vi "FileAscOpen.vi"(6 "提示语":refnum<vi>, 7 "Language":u32, 8 "进度条":refnum<vi>, 9 "进度数值":refnum<vi>, 10 "报文行数统计":refnum<vi>, 11 "file path (dialog if empty)":path caption="文件路径 （空时为对话框）") -> (0 "路径输出":path, 1 "重构的Data数组":u32[][](array[numeric]), 2 "统计数量":string[](array[string]), 3 "报文ID":string[](array[string]), 4 "基时间簇":T1 {"基时间秒" format="%#.6f"}, 5 "CAN报文统计":string[][](array[string]))   [LabVIEW 2015]
uses:
  <vilib>/Utility/file.llb/Read Delimited Spreadsheet (string).vi
  <vilib>/regexp/Match Regular Expression.xnode
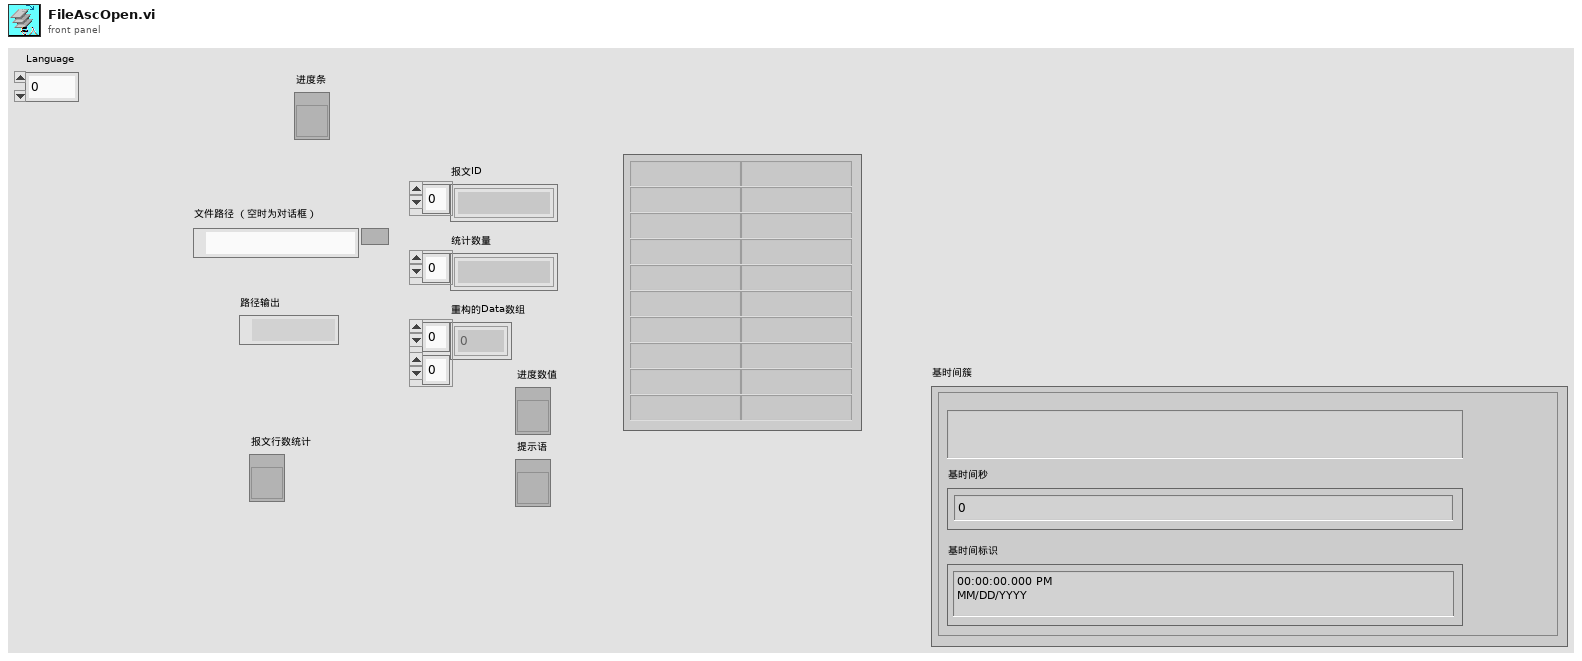
[diagram p1: front panel]
types:
  T1 = cluster{"基时间字符串":string, "基时间秒":dbl, "基时间标识":timestamp}
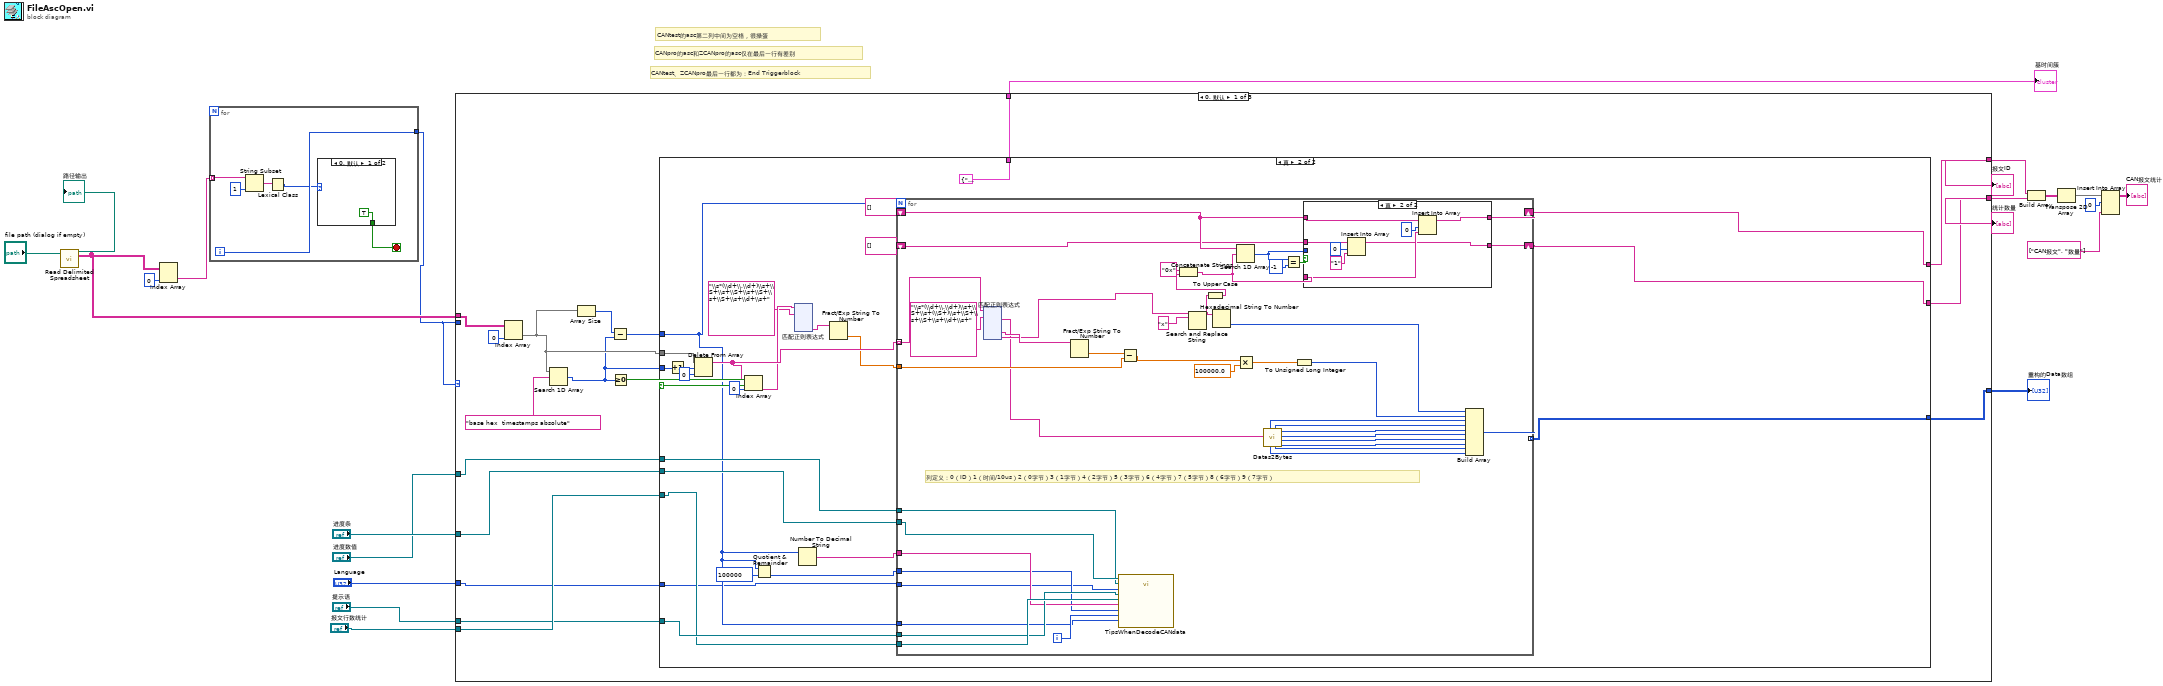
[diagram p0: block diagram]
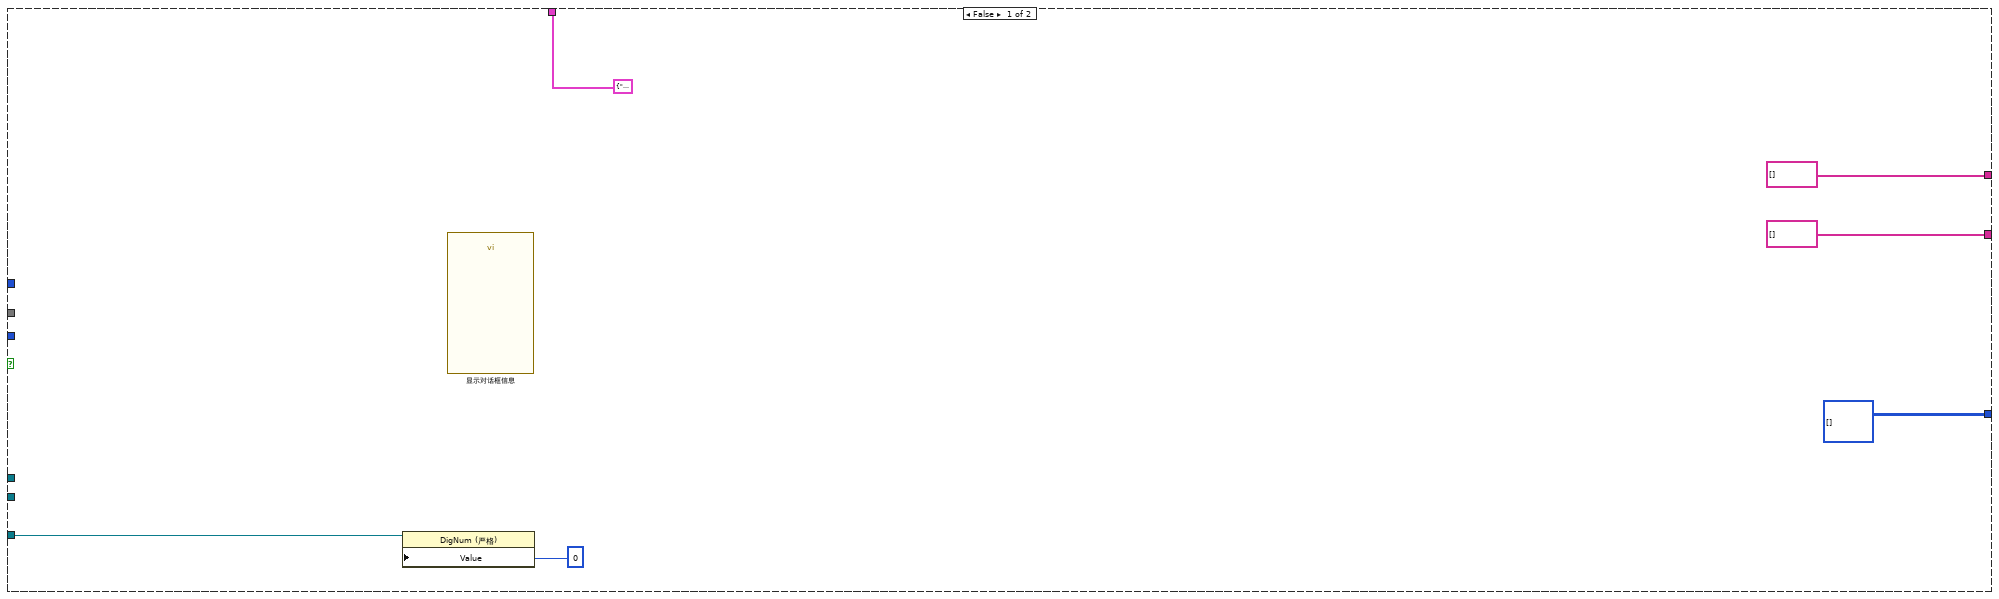
[diagram p2: hidden frame]
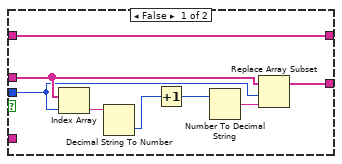
[diagram p3: hidden frame]
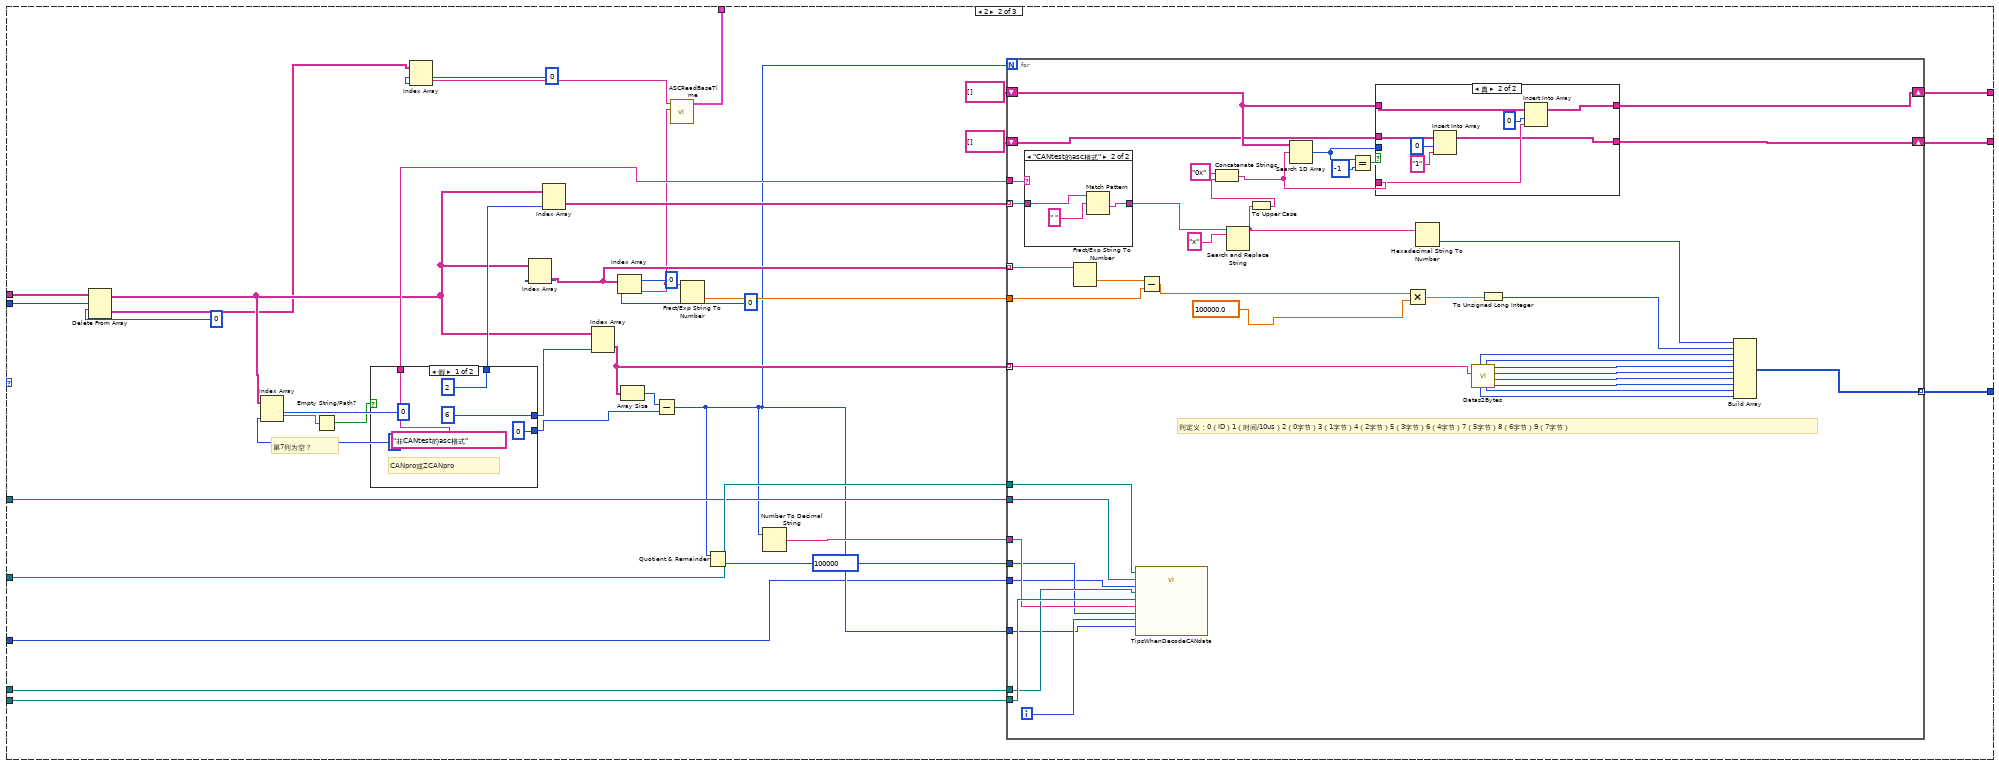
[diagram p4: hidden frame]
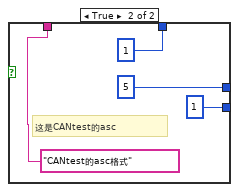
[diagram p5: hidden frame]
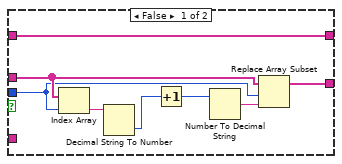
[diagram p7: hidden frame]
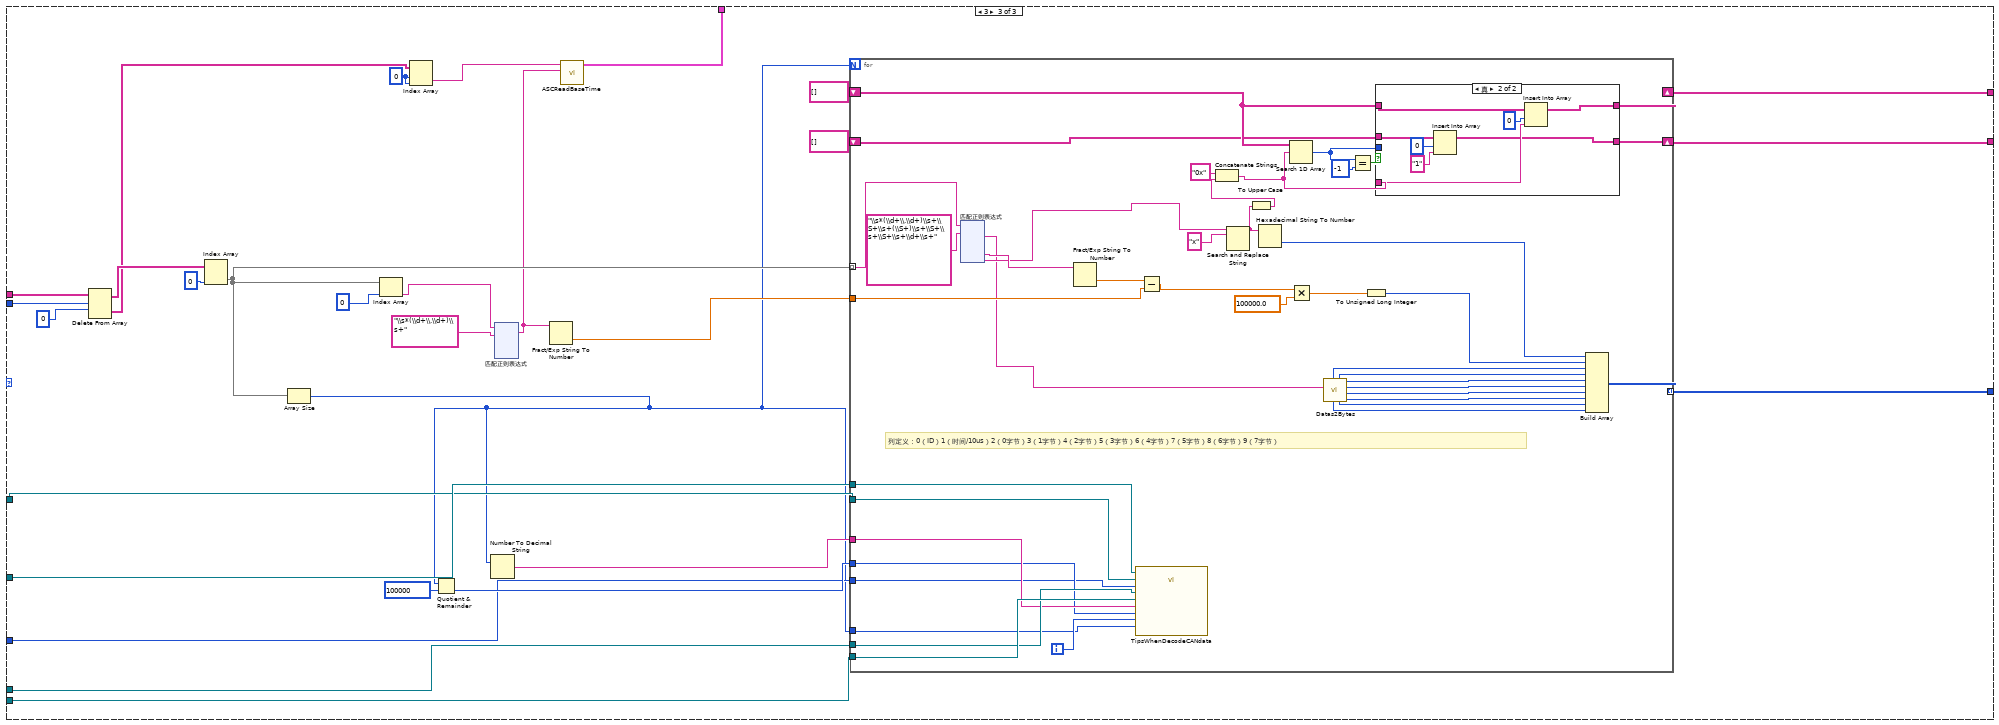
[diagram p8: hidden frame]
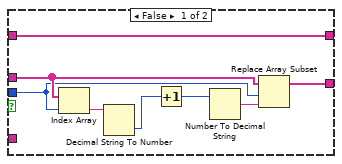
[diagram p9: hidden frame]
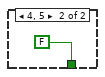
[diagram p10: hidden frame]
diagram:
  # "CANtest的asc第二列中间为空格，很操蛋"
  # "CANtest、ZCANpro最后一行都为：End Triggerblock"
  # "CANpro的asc和ZCANpro的asc仅在最后一行有差别"
  n1 = call-poly <vilib>:"Read Delimited Spreadsheet.vi"("file path (dialog if empty)"="file path (dialog if empty)") -> ("new file path (Not A Path if cancelled)"=→"路径输出":path, "all rows"=w5:string[][])  [unwired: 9 in, 4 out]
  n2 = Index Array(array=w5, index (col)=0 ("禁用的索引 (列)")) -> (element=w3:string[])  [unwired: 1 in]
  n3 = for {
    tunnel: w3 -> [w26] mode=indexing
    tunnel: [w23] -> w2
    i -> [w23]
    stop <- w24 stop-if-true
    n4 = String Subset(string=w26, length (rest)=1 ("长度（剩余）")) -> (substring=w22:string)  [unwired: 1 in]
    n5 = Lexical Class(1:w22) -> (0:w21:i16)
    n6 = case shown="0, 默认" w21 {
      tunnel: [TRUE FALSE] -> w24
      frame 0, Default {
      }
      frame 4, 5 {
      }
    }
  }
  n7 = case shown="0, 默认" w2 {
    tunnel: [w31 w405 w504] -> w20
    tunnel: [w29 w395 w498] -> w15
    tunnel: [w30 w394 w497] -> w14
    tunnel: "进度条" -> [w34 w393 w496]
    tunnel: "进度数值" -> [w35 w392 w495]
    tunnel: "提示语" -> [w33 w389 w492]
    tunnel: [w44 w372 w485] -> w8
    tunnel: "报文行数统计" -> [w45 w371 w484]
    tunnel: "Language" -> [w32 w370 w483]
    tunnel: w5 -> [w40 w369 w482]
    tunnel: w2 -> [_ w368 w481]
    frame 0, Default {
      n8 = Index Array(array=w40, index (col)=0 ("禁用的索引 (列)")) -> (element=w37:string[])  [unwired: 1 in]
      n9 = Search 1D Array(1D array=w37, element="base hex  timestamps absolute") -> (index of element=w36:i32)  [unwired: 1 in]
      n10 = Array Size(array=w37) -> (size(s)=w39:i32)
      n11 = Subtract(x=w39, y=w36) -> (x-y=w38:i32)
      n12 = Greater Or Equal To 0?(x=w36) -> (x >= 0?=w43:bool)
      n13 = case shown="真" w43 {
        tunnel: w45 -> [w50 w56]
        tunnel: [T1 {"基时间字符串"="", "基时间秒"=0.0, "基时间标识"=timestamp(0 s since 1904-01-01)} ("基时间簇") T1 {"基时间字符串"="", "基时间秒"=0.0, "基时间标识"=timestamp(0 s since 1904-01-01)} ("基时间簇")] -> w44
        tunnel: w38 -> [_ w58]
        tunnel: w37 -> [_ w76]
        tunnel: w36 -> [_ w74]
        tunnel: w35 -> [_ w62]
        tunnel: w34 -> [_ w63]
        tunnel: w33 -> [_ w61]
        tunnel: w32 -> [_ w55]
        tunnel: [u32[][] [] w52] -> w31
        tunnel: [string[] [] w53] -> w30
        tunnel: [string[] [] w54] -> w29
        frame False {
          n14 = property class="DigNum (严格)"(reference=w50, "Value"=0 ("值")) -> ()  [unwired: 1 in, 2 out]
          n15 = call "显示对话框信息"() -> ()  [unwired: 10 in, 2 out]
        }
        frame True {
          n16 = Increment(x=w74) -> (x+1=w75:i32)
          n17 = Delete From Array(array=w76, length=w75, index=0 ("索引")) -> (array with subset deleted=w68:string[])  [unwired: 1 out]
          n18 = Index Array(array=w68, index=0 ("索引")) -> (element=w67:string)
          n19 = Quotient & Remainder(x=w58, y=100000) -> (floor(x/y)=w57:i32)  [unwired: 1 out]
          n20 = xnode "匹配正则表达式"("输入字符串"=w67, "正则表达式"="\\s*(\\d+\\.\\d+)\\s+\\S+\\s+\\S+\\s+\\S+\\s+\\S+\\s+\\d+\\s+") -> ("子匹配 1"=w65:string)  [unwired: 4 in, 5 out]
          n21 = Number To Decimal String(number=w58) -> (decimal integer string=w59:string)  [unwired: 1 in]
          n22 = Fract/Exp String To Number(string=w65) -> (number=w64:dbl)  [unwired: 3 in, 1 out]
          n23 = for {
            N: w58 -> [_]
            tunnel: w68 -> [w210] mode=indexing
            tunnel: [w198] -> w52 mode=indexing
            shift-right: [w232] -> w54
            shift-left: string[] [] -> [w233]
            shift-right: [w228] -> w53
            shift-left: string[] [] -> [w229]
            tunnel: w58 -> [w213]
            tunnel: w63 -> [w194]
            tunnel: w57 -> [w212]
            tunnel: w61 -> [w215]
            tunnel: w59 -> [w214]
            tunnel: w64 -> [w225]
            tunnel: w56 -> [w216]
            tunnel: w55 -> [w211]
            tunnel: w62 -> [w193]
            i -> [w217]
            # "列定义：0（ID）1（时间/10us）2（0字节）3（1字节）4（2字节）5（3字节）6（4字节）7（5字节）8（6字节）9（7字节）"
            n24 = xnode "匹配正则表达式"("输入字符串"=w210, "正则表达式"="\\s*(\\d+\\.\\d+)\\s+\\S+\\s+(\\S+)\\s+\\S+\\s+\\S+\\s+\\d+\\s+") -> ("匹配之后"=w195:string, "子匹配 1"=w208:string, "子匹配 2"=w207:string)  [unwired: 4 in, 4 out]
            n25 = Fract/Exp String To Number(string=w208) -> (number=w226:dbl)  [unwired: 3 in, 1 out]
            n26 = call "TipsWhenDecodeCANdata.vi"("ProgressBar"=w194, "AllRowsNum"=w213, "i"=w217, "ProgressNum"=w193, "Language"=w211, "Tips"=w215, "MessageLinCnt"=w216, "txtAllRowsNum"=w214, "RowsLevel"=w212) -> ()  [unwired: 7 in]
            n27 = Subtract(x=w226, y=w225) -> (x-y=w224:dbl)
            n28 = Search and Replace String(input string=w207, search string="x" ("子字符串(\"\")")) -> (result string=w220:string)  [unwired: 6 in, 3 out]
            n29 = To Upper Case(1:w220) -> (0:w221:string)
            n30 = Concatenate Strings("0x" ("字符串"), w221) -> (w222:string)
            n31 = Hexadecimal String To Number(string=w220) -> (number=w197:u32)  [unwired: 2 in, 1 out]
            n32 = Search 1D Array(1D array=w233, element=w222) -> (index of element=w227:i32)  [unwired: 1 in]
            n33 = Multiply(x=w224, y=100000.0) -> (x*y=w234:dbl)
            n34 = call "Datas2Bytes.vi"("DATAs"=w195) -> ("Data5"=w201:u32, "Data4"=w202:u32, "Data3"=w203:u32, "Data2"=w204:u32, "Data6"=w200:u32, "Data1"=w205:u32, "Data7"=w199:u32, "Data0"=w206:u32)  [unwired: 3 in]
            n35 = Equal?(x=w227, y=-1) -> (x = y?=w230:bool)
            n36 = To Unsigned Long Integer(number=w234) -> (unsigned 32bit integer=w196:u32)
            n37 = case shown="真" w230 {
              tunnel: w233 -> [w359 w367]
              tunnel: [w359 w366] -> w232
              tunnel: w222 -> [_ w365]
              tunnel: w229 -> [w358 w362]
              tunnel: [w357 w363] -> w228
              tunnel: w227 -> [w352 _]
              frame False {
                n38 = Index Array(array=w358, index=w352) -> (element=w356:string)
                n39 = Decimal String To Number(string=w356) -> (number=w355:i32)  [unwired: 2 in, 1 out]
                n40 = Increment(x=w355) -> (x+1=w353:i32)
                n41 = Number To Decimal String(number=w353) -> (decimal integer string=w354:string)  [unwired: 1 in]
                n42 = Replace Array Subset(array=w358, new element=w354, index=w352) -> (w357:string[])
              }
              frame True {
                n43 = Insert Into Array(array=w362, index=0 ("索引"), new element="1" ("新元素/子数组")) -> (w363:string[])
                n44 = Insert Into Array(array=w367, index=0 ("索引"), new element=w365) -> (w366:string[])
              }
            }
            n45 = Build Array(w197, w196, w206, w205, w204, w203, w202, w201, w200, w199) -> (w198:u32[])
          }
        }
      }
    }
    frame 2 {
      w376 = 0 ("索引 (行)")
      # "第7列为空？"
      n46 = Delete From Array(array=w369, length=w368, index (row)=0 ("索引 (行)")) -> (deleted portion=w375:string[][], array with subset deleted=w381:string[][])  [unwired: 1 in]
      n47 = Index Array(array=w381, index (row)=0 ("索引 (行)"), index (col)=6 ("y")) -> (element=w382:string)
      n48 = Empty String/Path?(string/path=w382) -> (empty?=w380:bool)
      n49 = case shown="假" w380 {
        tunnel: [2 ("禁用的索引 (列)") 1 ("禁用的索引 (列)")] -> w403
        tunnel: [6 ("禁用的索引 (列)") 5 ("禁用的索引 (列)")] -> w398
        tunnel: ["非CANtest的asc格式" "CANtest的asc格式"] -> w385
        tunnel: [0 1] -> w379
        frame False {
          # "CANpro或ZCANpro"
        }
        frame True {
          # "这是CANtest的asc"
        }
      }
      n50 = Index Array(array=w375, index (row)=w376, index (col)=w376) -> (element=w374:string)
      n51 = Index Array(array=w381, index (col)=0 ("禁用的索引 (列)")) -> (element=w400:string[])  [unwired: 1 in]
      n52 = Index Array(array=w381, index (col)=w403) -> (element=w404:string[])  [unwired: 1 in]
      n53 = Index Array(array=w381, index (col)=w398) -> (element=w386:string[])  [unwired: 1 in]
      n54 = Index Array(array=w400, index=0 ("索引")) -> (element=w373:string)
      n55 = Array Size(array=w386) -> (size(s)=w378:i32)
      n56 = Subtract(x=w378, y=w379) -> (x-y=w377:i32)
      n57 = call "ASCReadBaseTime.vi"("偏置时间"=w373, "ASC首行"=w374) -> ("基时间簇"=w372:T1)  [unwired: 9 in]
      n58 = Fract/Exp String To Number(string=w373) -> (number=w387:dbl)  [unwired: 3 in, 1 out]
      n59 = Quotient & Remainder(x=w377, y=100000) -> (floor(x/y)=w390:i32)  [unwired: 1 out]
      n60 = Number To Decimal String(number=w377) -> (decimal integer string=w388:string)  [unwired: 1 in]
      n61 = for {
        N: w377 -> [_]
        tunnel: w400 -> [w447] mode=indexing
        tunnel: w386 -> [w414] mode=indexing
        tunnel: [w417] -> w405 mode=indexing
        shift-right: [w453] -> w395
        shift-left: string[] [] -> [w454]
        shift-right: [w449] -> w394
        shift-left: string[] [] -> [w450]
        tunnel: w404 -> [w436] mode=indexing
        tunnel: w377 -> [w430]
        tunnel: w393 -> [w426]
        tunnel: w392 -> [w427]
        tunnel: w390 -> [w429]
        tunnel: w389 -> [w432]
        tunnel: w388 -> [w431]
        tunnel: w387 -> [w445]
        tunnel: w385 -> [w437]
        tunnel: w371 -> [w433]
        tunnel: w370 -> [w428]
        i -> [w434]
        # "列定义：0（ID）1（时间/10us）2（0字节）3（1字节）4（2字节）5（3字节）6（4字节）7（5字节）8（6字节）9（7字节）"
        n62 = case shown="\"CANtest的asc格式\"" w437 {
          tunnel: w436 -> [w456 w459]
          tunnel: [w456 w458] -> w435
          frame "非CANtest的asc格式", Default {
          }
          frame "CANtest的asc格式" {
            n63 = Match Pattern(string=w459, regular expression=" " ("正则表达式")) -> (after substring=w458:string)  [unwired: 1 in, 3 out]
          }
        }
        n64 = Fract/Exp String To Number(string=w447) -> (number=w446:dbl)  [unwired: 3 in, 1 out]
        n65 = call "TipsWhenDecodeCANdata.vi"("ProgressBar"=w426, "AllRowsNum"=w430, "i"=w434, "ProgressNum"=w427, "Language"=w428, "Tips"=w432, "MessageLinCnt"=w433, "txtAllRowsNum"=w431, "RowsLevel"=w429) -> ()  [unwired: 7 in]
        n66 = Subtract(x=w446, y=w445) -> (x-y=w444:dbl)
        n67 = Search and Replace String(input string=w435, search string="x" ("子字符串(\"\")")) -> (result string=w440:string)  [unwired: 6 in, 3 out]
        n68 = To Upper Case(1:w440) -> (0:w441:string)
        n69 = Concatenate Strings("0x" ("字符串"), w441) -> (w442:string)
        n70 = Search 1D Array(1D array=w454, element=w442) -> (index of element=w448:i32)  [unwired: 1 in]
        n71 = Equal?(x=w448, y=-1) -> (x = y?=w451:bool)
        n72 = case shown="真" w451 {
          tunnel: w454 -> [w467 w475]
          tunnel: [w467 w474] -> w453
          tunnel: w442 -> [_ w473]
          tunnel: w450 -> [w466 w470]
          tunnel: [w465 w471] -> w449
          tunnel: w448 -> [w460 _]
          frame False {
            n73 = Index Array(array=w466, index=w460) -> (element=w464:string)
            n74 = Decimal String To Number(string=w464) -> (number=w463:i32)  [unwired: 2 in, 1 out]
            n75 = Increment(x=w463) -> (x+1=w461:i32)
            n76 = Number To Decimal String(number=w461) -> (decimal integer string=w462:string)  [unwired: 1 in]
            n77 = Replace Array Subset(array=w466, new element=w462, index=w460) -> (w465:string[])
          }
          frame True {
            n78 = Insert Into Array(array=w470, index=0 ("索引"), new element="1" ("新元素/子数组")) -> (w471:string[])
            n79 = Insert Into Array(array=w475, index=0 ("索引"), new element=w473) -> (w474:string[])
          }
        }
        n80 = Multiply(x=w444, y=100000.0) -> (x*y=w455:dbl)
        n81 = Hexadecimal String To Number(string=w440) -> (number=w416:u32)  [unwired: 2 in, 1 out]
        n82 = call "Datas2Bytes.vi"("DATAs"=w414) -> ("Data5"=w420:u32, "Data4"=w421:u32, "Data3"=w422:u32, "Data2"=w423:u32, "Data6"=w419:u32, "Data1"=w424:u32, "Data7"=w418:u32, "Data0"=w425:u32)  [unwired: 3 in]
        n83 = To Unsigned Long Integer(number=w455) -> (unsigned 32bit integer=w415:u32)
        n84 = Build Array(w416, w415, w425, w424, w423, w422, w421, w420, w419, w418) -> (w417:u32[])
      }
    }
    frame 3 {
      w488 = 0 ("索引 (行)")
      n85 = Delete From Array(array=w482, length=w481, index (row)=0 ("索引 (行)")) -> (deleted portion=w487:string[][], array with subset deleted=w489:string[][])  [unwired: 1 in]
      n86 = Index Array(array=w489, index (col)=0 ("禁用的索引 (列)")) -> (element=w480:string[])  [unwired: 1 in]
      n87 = Array Size(array=w480) -> (size(s)=w479:i32)
      n88 = Index Array(array=w480, index=0 ("索引")) -> (element=w478:string)
      n89 = Index Array(array=w487, index (row)=w488, index (col)=w488) -> (element=w486:string)
      n90 = Quotient & Remainder(x=w479, y=100000) -> (floor(x/y)=w493:i32)  [unwired: 1 out]
      n91 = Number To Decimal String(number=w479) -> (decimal integer string=w491:string)  [unwired: 1 in]
      n92 = xnode "匹配正则表达式"("输入字符串"=w478, "正则表达式"="\\s*(\\d+\\.\\d+)\\s+") -> ("所有匹配"=w476:string)  [unwired: 4 in, 5 out]
      n93 = Fract/Exp String To Number(string=w476) -> (number=w490:dbl)  [unwired: 3 in, 1 out]
      n94 = call "ASCReadBaseTime.vi"("偏置时间"=w476, "ASC首行"=w486) -> ("基时间簇"=w485:T1)  [unwired: 9 in]
      n95 = for {
        N: w479 -> [_]
        tunnel: w480 -> [w636] mode=indexing
        tunnel: [w624] -> w504 mode=indexing
        shift-right: [w660] -> w498
        shift-left: string[] [] -> [w661]
        shift-right: [w656] -> w497
        shift-left: string[] [] -> [w657]
        tunnel: w479 -> [w641]
        tunnel: w496 -> [w637]
        tunnel: w495 -> [w638]
        tunnel: w493 -> [w640]
        tunnel: w492 -> [w643]
        tunnel: w491 -> [w642]
        tunnel: w490 -> [w653]
        tunnel: w484 -> [w644]
        tunnel: w483 -> [w639]
        i -> [w645]
        # "列定义：0（ID）1（时间/10us）2（0字节）3（1字节）4（2字节）5（3字节）6（4字节）7（5字节）8（6字节）9（7字节）"
        n96 = xnode "匹配正则表达式"("输入字符串"=w636, "正则表达式"="\\s*(\\d+\\.\\d+)\\s+\\S+\\s+(\\S+)\\s+\\S+\\s+\\S+\\s+\\d+\\s+") -> ("匹配之后"=w621:string, "子匹配 1"=w634:string, "子匹配 2"=w633:string)  [unwired: 4 in, 4 out]
        n97 = Fract/Exp String To Number(string=w634) -> (number=w654:dbl)  [unwired: 3 in, 1 out]
        n98 = call "TipsWhenDecodeCANdata.vi"("ProgressBar"=w637, "AllRowsNum"=w641, "i"=w645, "ProgressNum"=w638, "Language"=w639, "Tips"=w643, "MessageLinCnt"=w644, "txtAllRowsNum"=w642, "RowsLevel"=w640) -> ()  [unwired: 7 in]
        n99 = Subtract(x=w654, y=w653) -> (x-y=w652:dbl)
        n100 = Search and Replace String(input string=w633, search string="x" ("子字符串(\"\")")) -> (result string=w648:string)  [unwired: 6 in, 3 out]
        n101 = To Upper Case(1:w648) -> (0:w649:string)
        n102 = Concatenate Strings("0x" ("字符串"), w649) -> (w650:string)
        n103 = Hexadecimal String To Number(string=w648) -> (number=w623:u32)  [unwired: 2 in, 1 out]
        n104 = Search 1D Array(1D array=w661, element=w650) -> (index of element=w655:i32)  [unwired: 1 in]
        n105 = Multiply(x=w652, y=100000.0) -> (x*y=w662:dbl)
        n106 = call "Datas2Bytes.vi"("DATAs"=w621) -> ("Data5"=w627:u32, "Data4"=w628:u32, "Data3"=w629:u32, "Data2"=w630:u32, "Data6"=w626:u32, "Data1"=w631:u32, "Data7"=w625:u32, "Data0"=w632:u32)  [unwired: 3 in]
        n107 = Equal?(x=w655, y=-1) -> (x = y?=w658:bool)
        n108 = To Unsigned Long Integer(number=w662) -> (unsigned 32bit integer=w622:u32)
        n109 = case shown="真" w658 {
          tunnel: w661 -> [w787 w795]
          tunnel: [w787 w794] -> w660
          tunnel: w650 -> [_ w793]
          tunnel: w657 -> [w786 w790]
          tunnel: [w785 w791] -> w656
          tunnel: w655 -> [w780 _]
          frame False {
            n110 = Index Array(array=w786, index=w780) -> (element=w784:string)
            n111 = Decimal String To Number(string=w784) -> (number=w783:i32)  [unwired: 2 in, 1 out]
            n112 = Increment(x=w783) -> (x+1=w781:i32)
            n113 = Number To Decimal String(number=w781) -> (decimal integer string=w782:string)  [unwired: 1 in]
            n114 = Replace Array Subset(array=w786, new element=w782, index=w780) -> (w785:string[])
          }
          frame True {
            n115 = Insert Into Array(array=w790, index=0 ("索引"), new element="1" ("新元素/子数组")) -> (w791:string[])
            n116 = Insert Into Array(array=w795, index=0 ("索引"), new element=w793) -> (w794:string[])
          }
        }
        n117 = Build Array(w623, w622, w632, w631, w630, w629, w628, w627, w626, w625) -> (w624:u32[])
      }
    }
  }
  "重构的Data数组" <- w20
  "报文ID" <- w15
  "统计数量" <- w14
  "基时间簇" <- w8
  n118 = Build Array(w15, w14) -> (w19:string[][])
  n119 = Transpose 2D Array(2D array=w19) -> (transposed array=w18:string[][])
  n120 = Insert Into Array(array=w18, index (row)=0 ("索引 (行)"), new element=string[] ["CAN报文", "数量"]) -> (→"CAN报文统计":string[][])  [unwired: 1 in]
